vi "Do.vi"(8 "error in (no error)":errorcluster, 10 "Actor in":refnum<class "Actor.lvclass">, 11 "Log Status":refnum<class "Log Status.lvclass">) -> (0 "error out":errorcluster, 2 "Actor out":refnum<class "Actor.lvclass">)   [LabVIEW 2016, in "Controller Actor.lvlib" / "Log Status.lvclass"]
uses:
  <userlib>/Common Components/Controller/Messages/Log Status/Log Status.lvclass
  <vilib>/ActorFramework/Actor/Actor.lvclass
  <userlib>/Common Components/Controller/Controller.lvclass
  C:/Program Files (x86)/National Instruments/LabVIEW 2016/vi.lib/ActorFramework/Actor/Actor.lvclass
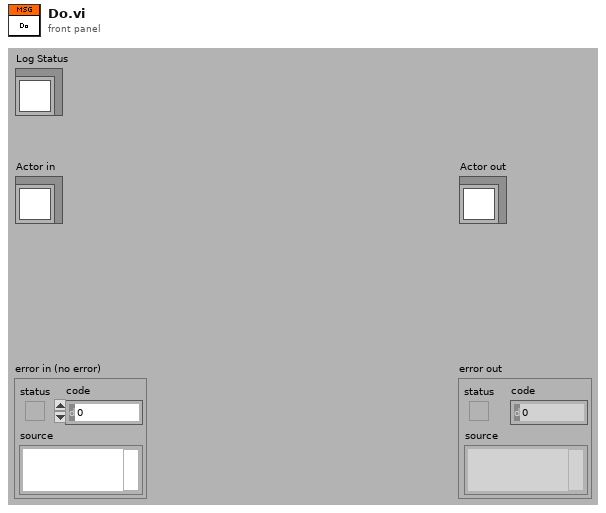
[diagram p1: front panel]
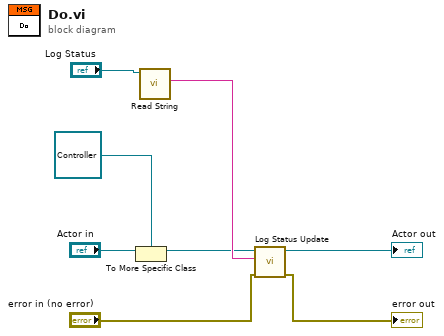
[diagram p0: block diagram]
diagram:
  n1 = To More Specific Class(target class=refnum<class "Controller.lvclass"> refnum ("Controller.lvclass"), reference="Actor in") -> (specific class reference=w4:refnum<class "Controller.lvclass">)  [unwired: 1 in, 1 out]
  n2 = call <userlib>:"Read String.vi"("Log Status in"="Log Status") -> ("String"=w5:string)  [unwired: 8 in, 2 out]
  n3 = call-dynamic "Log Status Update.vi"("error in (no error)"="error in (no error)", "String"=w5, "Controller in"=w4) -> ("error out"=→"error out":errorcluster, "Controller out"=→"Actor out":refnum<class "Controller.lvclass">)  [unwired: 7 in]
